vi "Group Data and Triggers for Display 20221121.vi"(7 "Chan":i32, 9 "scaling coefficients":T3[](array[typedef]), 10 "TrigCfg":T2(array[cluster]), 11 "Data waveform":T1(array[cluster])) -> (3 "Data for Display":T1(array[cluster]))   [LabVIEW 2021]
doc: "Sort and group Acquisition Data and thresholds. This preps for chart display.\n\nNote that this only works with one channel."
uses:
  <instrlib>/_niInstr/Multirecord Acquisition/Interface/v1/Host/Public/Scaling Coefficient.ctl
  <instrlib>/_niInstr/Multirecord Acquisition/Interface/v1/Host/niInstr Multirecord Acquisition v1 Host.lvclass
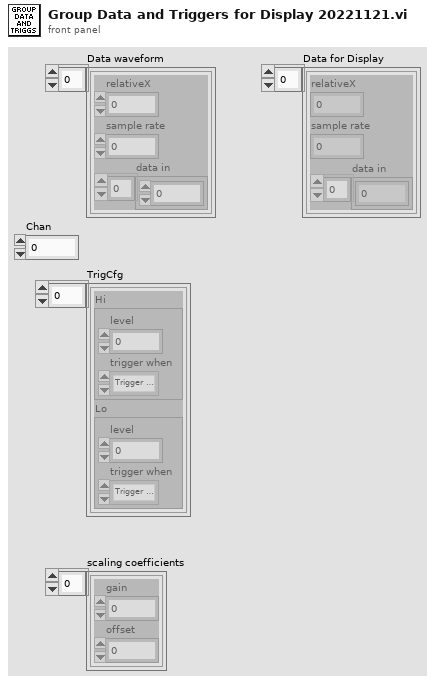
[diagram p1: front panel]
types:
  T1 = cluster{"relativeX":dbl, "sample rate":dbl, "data in":dbl[]}[]
  T2 = cluster{"Hi":cluster{"level":fxp<+/-,18,1>, "trigger when":enum8{"Trigger Above", "Trigger Below"}}, "Lo":cluster{"level":fxp<+/-,18,1>, "trigger when":enum8{"Trigger Above", "Trigger Below"}}}[]
  T3 = typedef "niInstr Multirecord Acquisition v1 Host.lvclass/Scaling Coefficient.ctl" = cluster{"gain":dbl, "offset":dbl}
  T4 = cluster{"Hi":cluster{"level":fxp<+/-,18,1>, "trigger when":enum8{"Trigger Above", "Trigger Below"}}, "Lo":cluster{"level":fxp<+/-,18,1>, "trigger when":enum8{"Trigger Above", "Trigger Below"}}}
  T5 = cluster{"relativeX":dbl, "sample rate":dbl, "data in":dbl[]}
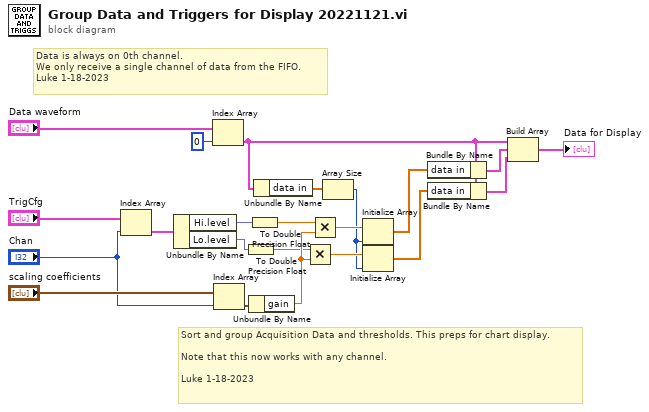
[diagram p0: block diagram]
diagram:
  # "Data is always on 0th channel.\nWe only receive a single channel of data from the FIFO.\nLuke 1-18-2023"
  # "Sort and group Acquisition Data and thresholds. This preps for chart display.\n\nNote that this now works with any channel.\n\nLuke 1-18-2023"
  n1 = Index Array(array="TrigCfg", index="Chan") -> (element=w3:T4)
  n2 = Unbundle By Name(w3) -> ("Hi.level"=w9:fxp<+/-,18,1>, "Lo.level"=w12:fxp<+/-,18,1>)
  n3 = Index Array(array="Data waveform", index=0) -> (element=w10:T5)
  n4 = Index Array(array="scaling coefficients", index="Chan") -> (element=w19:T3)
  n5 = To Double Precision Float(number=w12) -> (double precision float=w15:dbl)
  n6 = Unbundle By Name(w19) -> ("gain"=w22:dbl)
  n7 = To Double Precision Float(number=w9) -> (double precision float=w14:dbl)
  n8 = Unbundle By Name(w10) -> ("data in"=w11:dbl[])
  n9 = Multiply(x=w15, y=w22) -> (x*y=w21:dbl)
  n10 = Multiply(x=w14, y=w22) -> (x*y=w20:dbl)
  n11 = Array Size(array=w11) -> (size(s)=w13:i32)
  n12 = Initialize Array(w20, w13) -> (w16:dbl[])
  n13 = Initialize Array(w21, w13) -> (w17:dbl[])
  n14 = Bundle By Name(cluster=w10, "data in"=w16) -> (w6:T5)
  n15 = Bundle By Name(cluster=w10, "data in"=w17) -> (w7:T5)
  n16 = Build Array(w10, w6, w7) -> (→"Data for Display":T1)
